vi "Create All Message Queues.vi"(8 "error in (no error)":errorcluster) -> (0 "error out":errorcluster, 3 "Message Queues out":T1)   [LabVIEW 2018, in "HOG Message Queue.lvlib"]
doc: "This VI creates and initializes all the message queues for your application. If your application requires more than one message queue, right-click the \"Message Queues\" constant above and select Open Type Def. Add the new Message Queue(s) to the type definition, then initialize them in this VI."
uses:
  HOG Message Queue.lvlib
  All Message Queues.ctl
  Message Cluster.ctl
  Enqueue Message (Single).vi
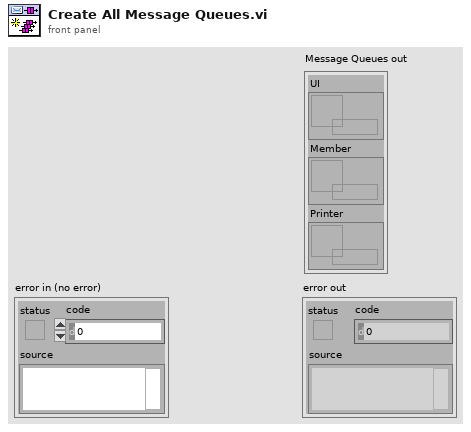
[diagram p1: front panel]
types:
  T1 = typedef "HOG Message Queue.lvlib/All Message Queues.ctl" = cluster{"UI":refnum<queue>, "Member":refnum<queue>, "Printer":refnum<queue>}
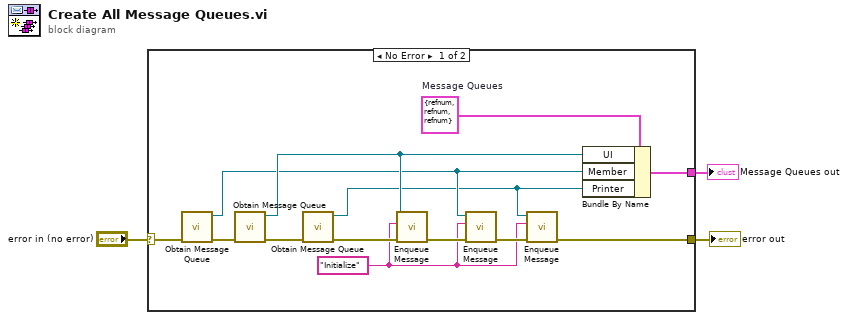
[diagram p0: block diagram]
diagram:
  n1 = case shown="No Error" "error in (no error)" {
    selector: "error in (no error)" -> [w13 w17]
    tunnel: [w6 w17] -> w3
    tunnel: [w15 _] -> w2
    frame No Error {
      w4 = "Initialize" ("Message")
      w16 = T1 {"UI"=refnum, "Member"=refnum, "Printer"=refnum}  # Message Queues
      n2 = call "Obtain Message Queue.vi"("error in (no error)"=w13) -> ("error out"=w12:errorcluster, "Message Queue"=w10:refnum<queue>)  [unwired: 9 in]
      n3 = call "Obtain Message Queue.vi"("error in (no error)"=w12) -> ("error out"=w9:errorcluster, "Message Queue"=w14:refnum<queue>)  [unwired: 9 in]
      n4 = call "Obtain Message Queue.vi"("error in (no error)"=w9) -> ("error out"=w8:errorcluster, "Message Queue"=w5:refnum<queue>)  [unwired: 9 in]
      n5 = call-poly "Enqueue Message.vi"("error in (no error)"=w8, "Message"=w4, "Message Queue"=w14) -> ("error out"=w11:errorcluster)  [unwired: 7 in, 1 out]
      n6 = call-poly "Enqueue Message.vi"("error in (no error)"=w11, "Message"=w4, "Message Queue"=w10) -> ("error out"=w7:errorcluster)  [unwired: 7 in, 1 out]
      n7 = call-poly "Enqueue Message.vi"("error in (no error)"=w7, "Message"=w4, "Message Queue"=w5) -> ("error out"=w6:errorcluster)  [unwired: 7 in, 1 out]
      n8 = Bundle By Name(cluster=w16, "UI"=w14, "Member"=w10, "Printer"=w5) -> (w15:T1)
    }
    frame Error {
    }
  }
  "Message Queues out" <- w2
  "error out" <- w3
